vi "Framework.Create.Plugins.vi"(8 "error in (no error)":errorcluster, 10 "Plugin Configurations":refnum<class "Plugin Configuration.lvclass">[](array[class]), 11 "Framework in":refnum<class "Framework.lvclass">) -> (0 "error out":errorcluster, 2 "Plugins":refnum<class "Plugin.lvclass">[](array[class]), 3 "Framework out":refnum<class "Framework.lvclass">)   [LabVIEW 2017, in "DSF Core.lvlib" / "Framework.lvclass"]
uses:
  Framework.lvclass
  Shared/Classes/Plugin/Plugin Configuration.lvclass
  Plugin/Plugin.lvclass
  Shared/Classes/Plugin/Plugin Configuration.lvclass/Plugin Configuration.ctl
  Framework.lvclass/Framework.ctl
  Component Loader/Component Loader.lvclass
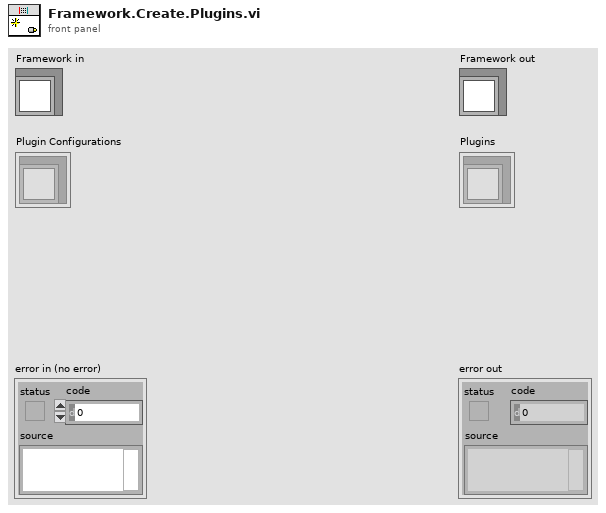
[diagram p1: front panel]
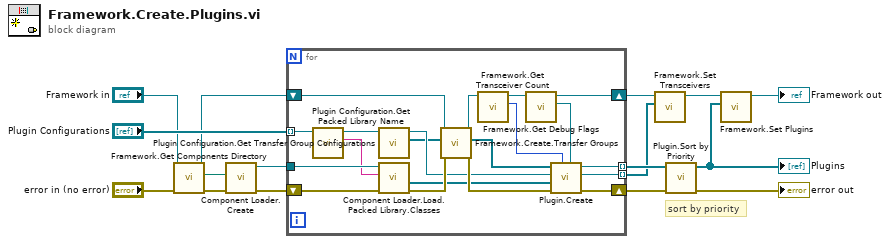
[diagram p0: block diagram]
diagram:
  # "sort by priority"
  n1 = call "Framework.Get Components Directory.vi"("error in (no error)"="error in (no error)", "Framework in"="Framework in") -> ("error out"=w4:errorcluster, "components directory"=w5:path, "Framework out"=w7:refnum<class "Framework.lvclass">)  [unwired: 7 in]
  n2 = call "Component Loader.Create.vi"("error in (no error)"=w4, "components directory"=w5) -> ("error out"=w1:errorcluster, "Component Loader out"=w3:refnum<class "Component Loader.lvclass">)  [unwired: 8 in]
  n3 = for {
    shift-right: [w34] -> w15
    shift-left: w1 -> [w19]
    shift-right: [w30] -> w11
    shift-left: w7 -> [w33]
    tunnel: "Plugin Configurations" -> [w28] mode=indexing
    tunnel: [w32] -> w13 mode=indexing
    tunnel: w3 -> [w26]
    tunnel: [w23] -> w2 mode=indexing
    n4 = call "Plugin Configuration.Get Packed Library Name.vi"("Plugin Configuration in"=w28) -> ("packed library name"=w25:string, "Plugin Configuration out"=w27:refnum<class "Plugin Configuration.lvclass">)  [unwired: 9 in]
    n5 = call "Plugin Configuration.Get Transfer Group Configurations.vi"("Plugin Configuration in"=w27) -> ("Transfer Group Configurations"=w17:refnum<class "Transfer Group Configuration.lvclass">[], "Plugin Configuration out"=w18:refnum<class "Plugin Configuration.lvclass">)  [unwired: 9 in]
    n6 = call "Component Loader.Load.Packed Library.Classes.vi"("error in (no error)"=w19, "packed library name"=w25, "Component Loader in"=w26) -> ("error out"=w35:errorcluster, "objects"=w21:refnum<class>[])  [unwired: 6 in, 1 out]
    n7 = call "Framework.Create.Transfer Groups.vi"("error in (no error)"=w35, "Transfer Group Configurations"=w17, "Framework in"=w33) -> ("error out"=w36:errorcluster, "Transfer Groups"=w20:refnum<class "Transfer Group.lvclass">[], "Framework out"=w31:refnum<class "Framework.lvclass">)  [unwired: 6 in]
    n8 = call "Framework.Get Transceiver Count.vi"("Framework in"=w31) -> ("transceiver count"=w24:i32, "Framework out"=w29:refnum<class "Framework.lvclass">)  [unwired: 9 in]
    n9 = call "Framework.Get Debug Flags.vi"("Framework in"=w29) -> ("Debug Flags"=w22:refnum<class "Debug Flags.lvclass">, "Framework out"=w30:refnum<class "Framework.lvclass">)  [unwired: 9 in]
    n10 = call "Plugin.Create.vi"("Debug Flags"=w22, "transceiver count"=w24, "error in (no error)"=w36, "component classes"=w21, "Plugin Configuration"=w18, "Transfer Groups"=w20) -> ("error out"=w34:errorcluster, "Transceiver"=w23:refnum<class "Transceiver.lvclass">, "Plugin out"=w32:refnum<class "Plugin.lvclass">)  [unwired: 3 in]
  }
  n11 = call "Framework.Set Transceivers.vi"("Transceivers"=w2, "Framework in"=w11) -> ("Framework out"=w10:refnum<class "Framework.lvclass">)  [unwired: 9 in]
  n12 = call "Plugin.Sort by Priority.vi"("error in (no error)"=w15, "Plugins in"=w13) -> ("error out"=→"error out":errorcluster, "Plugins out"=w12:refnum<class "Plugin.lvclass">[])  [unwired: 8 in]
  "Plugins" <- w12
  n13 = call "Framework.Set Plugins.vi"("Plugins"=w12, "Framework in"=w10) -> ("Framework out"=→"Framework out":refnum<class "Framework.lvclass">)  [unwired: 9 in]
